vi "Home.vi"() -> ()   [LabVIEW 2020]
panel:
  in  "Cancel Button":bool
  in  "PTPS":bool
  in  "SWPS":bool
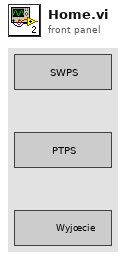
[diagram p1: front panel]
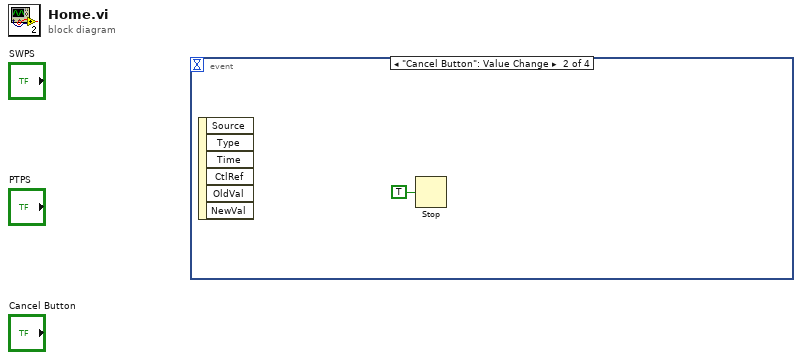
[diagram p0: block diagram]
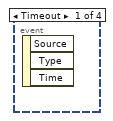
[diagram p2: hidden frame]
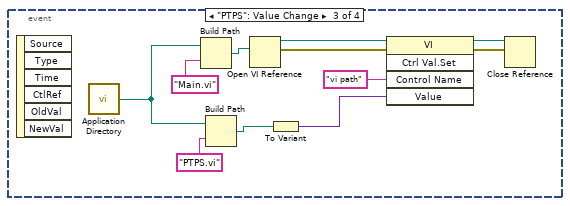
[diagram p3: hidden frame]
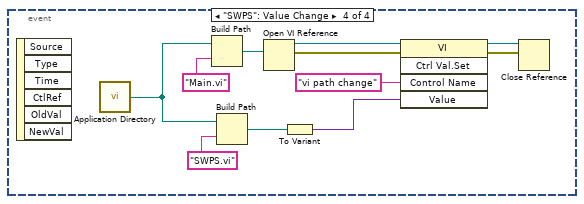
[diagram p4: hidden frame]
diagram:
  n1 = event shown="[1] \"Cancel Button\": Value Change" {
    selector: _ -> [_ _ _ _]
    dyn-events: _ -> [_ _ _ _]
    timeout: _ -> [_ _ _ _]
    event Timeout {
      n2 = event-data() -> ()  [unwired: 1 in, 3 out]
    }
    event "Cancel Button": Value Change {
      n3 = event-data() -> ()  [unwired: 1 in, 6 out]
      n4 = Stop(stop? (T)=TRUE) -> ()
    }
    event "PTPS": Value Change {
      n5 = event-data() -> ()  [unwired: 1 in, 6 out]
      n6 = call <vilib>:"Application Directory.vi"() -> ("Application Directory"=w4:path)
      n7 = Build Path(base path=w4, name or relative path="Main.vi") -> (appended path=w2:path)
      n8 = Build Path(base path=w4, name or relative path="PTPS.vi") -> (appended path=w3:path)
      n9 = Open VI Reference(vi path=w2) -> (vi reference=w10:refnum<vi>, error out=w9:errorcluster)  [unwired: 5 in]
      n10 = To Variant(anything=w3) -> (Variant=w7:variant)
      n11 = invoke class="VI" method="Ctrl Val.Set"(reference=w10, error in=w9, "Control Name"="vi path", "Value"=w7) -> (reference out=w11:refnum<vi>, error out=w12:errorcluster)  [unwired: 1 in, 3 out]
      n12 = Close Reference(reference=w11, error in (no error)=w12) -> ()  [unwired: 1 out]
    }
    event "SWPS": Value Change {
      n13 = event-data() -> ()  [unwired: 1 in, 6 out]
      n14 = call <vilib>:"Application Directory.vi"() -> ("Application Directory"=w13:path)
      n15 = Build Path(base path=w13, name or relative path="Main.vi") -> (appended path=w16:path)
      n16 = Build Path(base path=w13, name or relative path="SWPS.vi") -> (appended path=w14:path)
      n17 = Open VI Reference(vi path=w16) -> (vi reference=w21:refnum<vi>, error out=w20:errorcluster)  [unwired: 5 in]
      n18 = To Variant(anything=w14) -> (Variant=w18:variant)
      n19 = invoke class="VI" method="Ctrl Val.Set"(reference=w21, error in=w20, "Control Name"="vi path change", "Value"=w18) -> (reference out=w22:refnum<vi>, error out=w23:errorcluster)  [unwired: 1 in, 3 out]
      n20 = Close Reference(reference=w22, error in (no error)=w23) -> ()  [unwired: 1 out]
    }
  }
